vi "Value Change.vi"(8 "Settings In":T1={"Step Values"=[], "Only Execute When Test Running"=TRUE, "Reset Sequence When Test Starts"=TRUE, "Current Sequence ID"=0, "Total Iterations"=0, "Last Timestamp"=0.0, "Number of Sequence Steps"=0, "Num of Analog Channels"=0, "Num of Digital Channels"=0, "Delay Before Starting Sequence"=0.0, "Changed"=FALSE}, 9 "Tree Data":cluster{"Tag":string[], "Settings":T3[]} {"Settings"."Data Type" items=["Tree Parent"=-1, "Numeric"=0, "String"=1, "Boolean"=2, "Enum"=3]}, 10 "Tree Tag":string, 11 "Init Refs":T5) -> (0 "Settings Out":T1={"Step Values"=[], "Only Execute When Test Running"=TRUE, "Reset Sequence When Test Starts"=TRUE, "Current Sequence ID"=0, "Total Iterations"=0, "Last Timestamp"=0.0, "Number of Sequence Steps"=0, "Num of Analog Channels"=0, "Num of Digital Channels"=0, "Delay Before Starting Sequence"=0.0, "Changed"=FALSE}, 3 "Tree Data out":cluster{"Tag":string[], "Settings":T3[]} {"Settings"."Data Type" items=["Tree Parent"=-1, "Numeric"=0, "String"=1, "Boolean"=2, "Enum"=3]})   [LabVIEW 2020, in "Sequencer with Output Values.lvlib" / "Sequencer with Output Values.lvclass"]
uses:
  Sequencer with Output Values.lvclass
  Control Refs.ctl
  Tree Item Settings.ctl
  Data Type.ctl
  Params.ctl
  Step Settings.ctl
  Data Type Enum.ctl
  Global Tree Data.vi
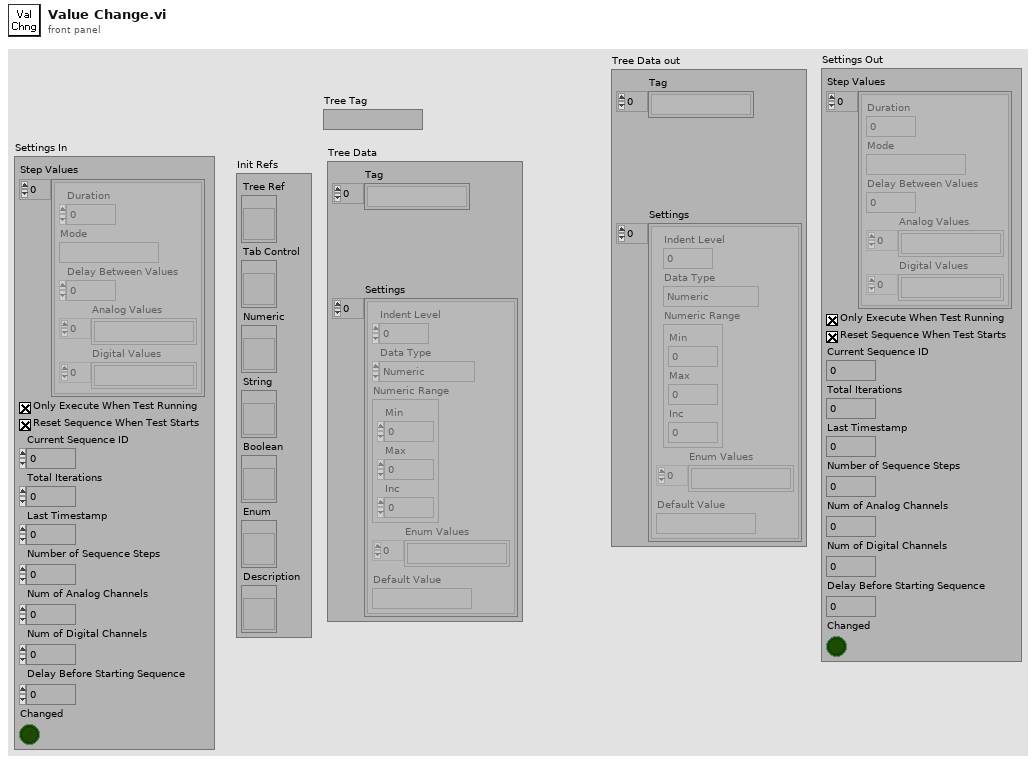
[diagram p1: front panel]
types:
  T1 = typedef "Sequencer with Output Values.lvlib/Sequencer with Output Values.lvclass/Params.ctl" = cluster{"Step Values":T2[], "Only Execute When Test Running":bool, "Reset Sequence When Test Starts":bool, "Current Sequence ID":u32, "Total Iterations":u32, "Last Timestamp":dbl, "Number of Sequence Steps":i32, "Num of Analog Channels":i32, "Num of Digital Channels":i32, "Delay Before Starting Sequence":dbl, "Changed":bool}
  T2 = typedef "Sequencer with Output Values.lvlib/Sequencer with Output Values.lvclass/Step Settings.ctl" = cluster{"Duration":dbl, "Mode":string, "Delay Between Values":dbl, "Analog Values":string[], "Digital Values":string[]}
  T3 = typedef "Sequencer with Output Values.lvlib/Sequencer with Output Values.lvclass/Tree Item Settings.ctl" = cluster{"Indent Level":i32, "Data Type":T4, "Numeric Range":cluster{"Min":dbl, "Max":dbl, "Inc":dbl}, "Enum Values":string[], "Default Value":string}
  T4 = typedef "Sequencer with Output Values.lvlib/Sequencer with Output Values.lvclass/Data Type.ctl" = i16
  T5 = typedef "Sequencer with Output Values.lvlib/Sequencer with Output Values.lvclass/Control Refs.ctl" = cluster{"Tree Ref":refnum<vi>, "Tab Control":refnum<vi>, "Numeric":refnum<vi>, "String":refnum<vi>, "Boolean":refnum<vi>, "Enum":refnum<vi>, "Description":refnum<vi>}
  T6 = typedef "Sequencer with Output Values.lvlib/Sequencer with Output Values.lvclass/Data Type Enum.ctl" = enum16{"Numeric", "String", "Boolean", "Enum"}
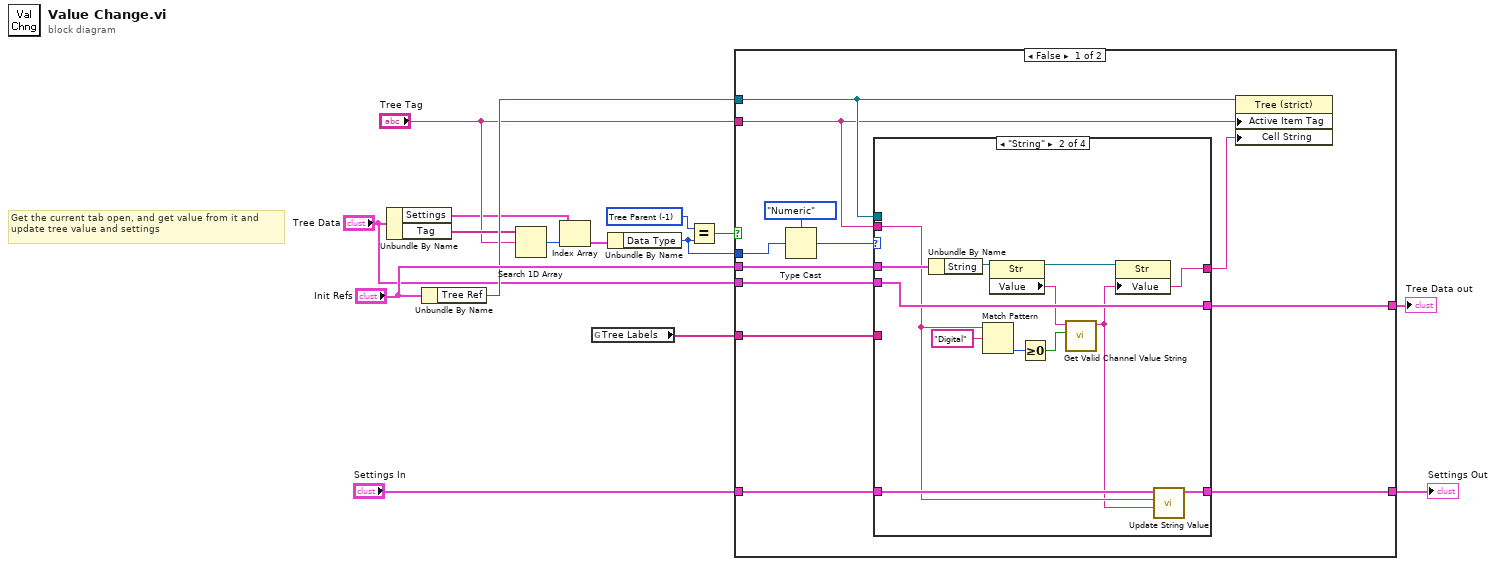
[diagram p0: block diagram]
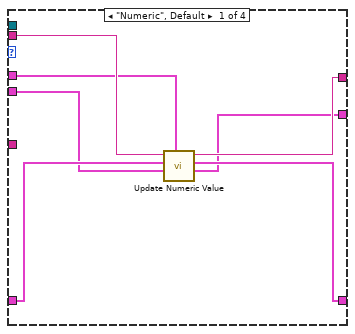
[diagram p2: hidden frame]
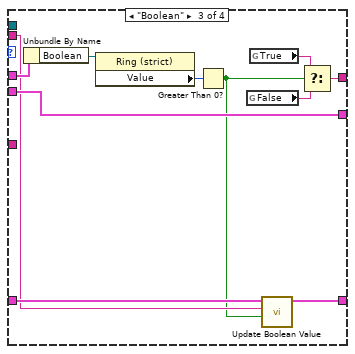
[diagram p3: hidden frame]
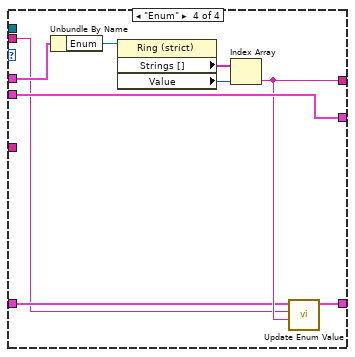
[diagram p4: hidden frame]
diagram:
  w8 = T4 -1 items=["Tree Parent"=-1, "Numeric"=0, "String"=1, "Boolean"=2, "Enum"=3, "Command"=4, "Numeric Min/Max"=5] ("Data Type")
  # "Get the current tab open, and get value from it and update tree value and settings"
  n1 = Unbundle By Name("Tree Data") -> ("Settings"=w11:T3[], "Tag"=w13:string[])
  n2 = Unbundle By Name("Init Refs") -> ("Tree Ref"=w14:refnum<vi>)
  n3 = Search 1D Array(1D array=w13, element="Tree Tag") -> (index of element=w10:i32)  [unwired: 1 in]
  n4 = Index Array(array=w11, index=w10) -> (element=w9:T3)
  n5 = global read "Global Tree Data.vi" "Tree Labels"() -> (w2:string[])
  n6 = Unbundle By Name(w9) -> ("Data Type"=w6:T4)
  n7 = Equal?(x=w8, y=w6) -> (x = y?=w7:bool)
  n8 = case shown="False" w7 {
    tunnel: "Init Refs" -> [w27 _]
    tunnel: w14 -> [w22 _]
    tunnel: "Tree Tag" -> [w21 _]
    tunnel: w6 -> [w26 _]
    tunnel: [w20 w68] -> w4
    tunnel: "Tree Data" -> [w19 w68]
    tunnel: "Settings In" -> [w18 w67]
    tunnel: w2 -> [w17 _]
    tunnel: [w16 w67] -> w1
    frame False {
      n9 = Type Cast(type=Data_Type_Enum."Numeric" ("Data Type"), x=w26) -> (*(type *) &x=w24:T6)
      n10 = case shown="\"String\"" w24 {
        tunnel: w27 -> [w31 w46 w57 w63]
        tunnel: [w34 w35 w55 w61] -> w23
        tunnel: w22 -> [_ _ _ _]
        tunnel: w21 -> [w33 w40 w48 w58]
        tunnel: [w28 w44 w53 w66] -> w20
        tunnel: w19 -> [w29 w44 w53 w66]
        tunnel: w18 -> [w30 w43 w50 w60]
        tunnel: w17 -> [_ _ _ _]
        tunnel: [w32 w42 w49 w59] -> w16
        frame "Numeric", Default {
          n11 = call "Update Numeric Value.vi"("Init Refs"=w31, "Tree Data in"=w29, "Settings In"=w30, "Tree Tag"=w33) -> ("Tree Data out"=w28:cluster{"Tag":string[], "Settings":T3[]}, "Settings In out"=w32:T1, "New Tree Value"=w34:string)  [unwired: 5 in]
        }
        frame "String" {
          n12 = Unbundle By Name(w46) -> ("String"=w45:refnum<vi>)
          n13 = Match Pattern(string=w40, regular expression="Digital") -> (offset past match=w38:i32)  [unwired: 1 in, 3 out]
          n14 = property class="Str"(reference=w45) -> (reference out=w36:refnum<vi>, "Value"=w41:string)  [unwired: 1 in, 1 out]
          n15 = Greater Or Equal To 0?(x=w38) -> (x >= 0?=w37:bool)
          n16 = call "Get Valid Channel Value String.vi"("Digital"=w37, "Channel Values"=w41) -> ("Valid Channel Values"=w35:string)  [unwired: 9 in]
          n17 = property class="Str"(reference=w36, "Value"=w35) -> ()  [unwired: 1 in, 2 out]
          n18 = call "Update String Value.vi"("Value"=w35, "Tree Tag"=w40, "Settings In"=w43) -> ("Settings Out"=w42:T1)  [unwired: 8 in]
        }
        frame "Boolean" {
          n19 = Unbundle By Name(w57) -> ("Boolean"=w56:refnum<vi>)
          n20 = property class="Ring (strict)"(reference=w56) -> ("Value"=w54:u16)  [unwired: 1 in, 2 out]
          n21 = Greater Than 0?(x=w54) -> (x > 0?=w47:bool)
          n22 = global read "Global Tree Data.vi" "False"() -> (w51:string)
          n23 = global read "Global Tree Data.vi" "True"() -> (w52:string)
          n24 = call "Update Boolean Value.vi"("Value"=w47, "Tree Tag"=w48, "Settings In"=w50) -> ("Settings Out"=w49:T1)  [unwired: 8 in]
          n25 = Select(t=w52, s=w47, f=w51) -> (s? t:f=w55:string)
        }
        frame "Enum" {
          n26 = Unbundle By Name(w63) -> ("Enum"=w62:refnum<vi>)
          n27 = property class="Ring (strict)"(reference=w62) -> ("Strings []"=w65:string[], "Value"=w64:u16)  [unwired: 1 in, 2 out]
          n28 = Index Array(array=w65, index=w64) -> (element=w61:string)
          n29 = call "Update Enum Value.vi"("Value"=w61, "Tree Tag"=w58, "Settings In"=w60) -> ("Settings Out"=w59:T1)  [unwired: 8 in]
        }
      }
      n30 = property class="Tree (strict)"(reference=w22, "Active Item Tag"=w21, "Cell String"=w23) -> ()  [unwired: 1 in, 2 out]
    }
    frame True {
    }
  }
  "Tree Data out" <- w4
  "Settings Out" <- w1
